vi "Init.vi"(8 "error in (no error)":errorcluster, 10 "Variant":variant, 11 "Avantes in":refnum<class "Avantes.lvclass">) -> (0 "error out":errorcluster, 3 "Avantes out":refnum<class "Avantes.lvclass">)   [LabVIEW 2020, in "Avantes.lvclass"]
uses:
  <instrlib>/Classes/CCD/Avantes/Avantes.lvclass
  <instrlib>/Classes/CCD/Avantes/Avantes.lvclass/Avantes.ctl
panel:
  out "Debug_Settings_Spectromter":string caption="Debug Spectromter"
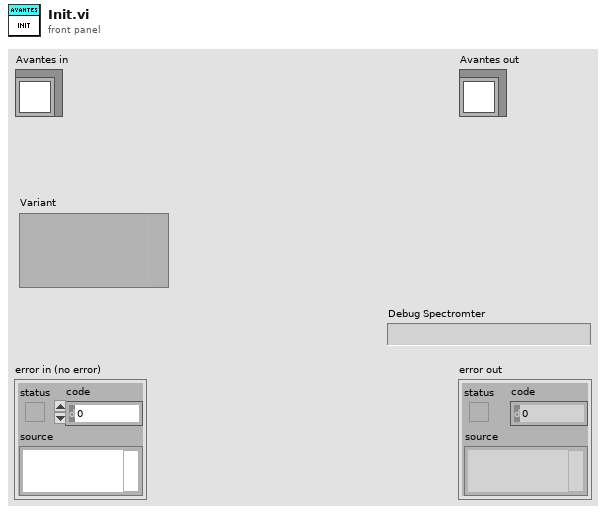
[diagram p1: front panel]
types:
  T1 = typedef "clusterdef.ctl" = cluster{"Len":u16, "ConfigVersion":u16, "UserFriendlyId":u8[], "DetectorType":cluster{"SensorType":u8, "NrPixels":u16, "Fit":sgl[], "NLEnable":u8, "NLCorrect":dbl[], "LowNLCounts":dbl, "HighNLCounts":dbl, "Gain":sgl[], "Reserved":sgl, "Offset":sgl[], "Extern Offset":sgl, "DefectivePixels":u16[]}, "IrradianceType":cluster{"SpectrumCalibrationType":cluster{"SmoothingType":cluster{"m_SmoothPix":u16, "SmoothModel":u8}, "CalInttime":sgl, "CalibConvers":sgl[]}, "CalibrationType":u8, "FiberDiameter":i32}, "SpectrumCalibrationType":cluster{"SmoothingType":cluster{"m_SmoothPix":u16, "SmoothModel":u8}, "CalInttime":sgl, "CalibConvers":sgl[]}, "SpectrumCorrectionType":sgl[], "StandAloneType":cluster{"StandAloneType":u8, "MeasConfigType":cluster{"StartPixel":u16, "StopPixel":u16, "IntegrationTime":sgl, "IntegrationDelay":u32, "NrAverages":u32, "DarkCorrectionType":cluster{"Enable CorDynDark":u8, "ForgetPercentage":u8}, "SmoothingType":cluster{"SmoothPix":u16, "SmoothModel":u8}, "SatDetection":u8, "TriggerType":cluster{"Trigger Mode":u8, "Trigger Source":u8, "Trigger SourceType":u8}, "ControlSettingsType":cluster{"StrobeControl":u16, "LaserDelay":u32, "LaserWidth":u32, "LaserWaveLength":sgl, "StoreToRam":u16}}, "Nmsr":i16}, "DynamicStorageType":cluster{"Nmsr":i32, "Reserved":u8[]}, "TempSensorType":sgl[], "TecControlType":cluster{"Enable":u8, "Setpoint":sgl, "Fit[NR_DAC_POL_COEF]":sgl[]}, "ProcessControlType":cluster{"AnalogLow":sgl[], "AnalogHigh":sgl[], "DigitalLow":sgl[], "DigitalHigh":sgl[]}, "EthernetSettingsType":cluster{"IpAddr":u32, "NetMask":u32, "Gateway":u32, "DhcpEnabled":u8, "TcpPort":u16, "LinkStatus":u8}, "Reserved":u8[], "OemData":u8[]}
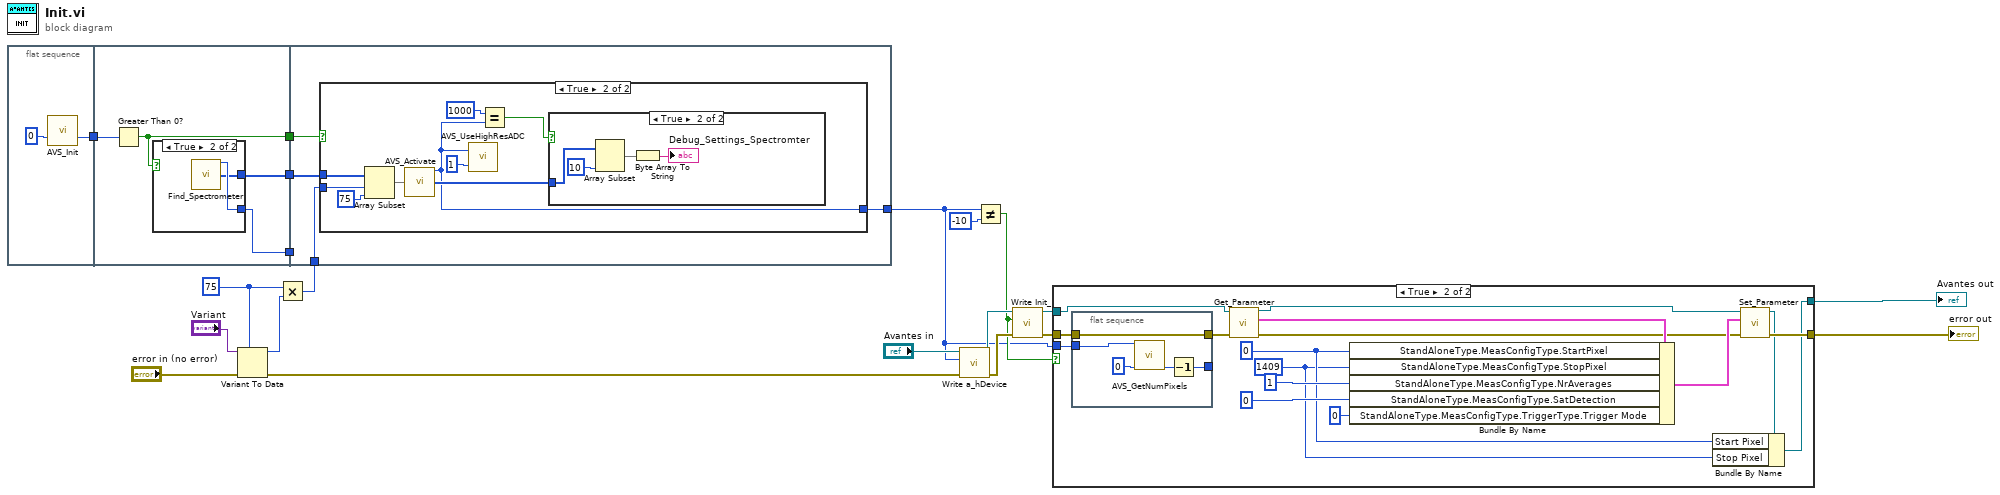
[diagram p0: block diagram]
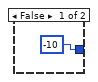
[diagram p4: hidden frame]
diagram:
  w11 = 75 ("length")
  n1 = flat-sequence {
    tunnel: [w21] -> w20
    tunnel: w20 -> [w26]
    tunnel: [w25] -> w19
    tunnel: [w24] -> w18
    tunnel: [w23] -> w17
    tunnel: w19 -> [_]
    tunnel: w18 -> [w32]
    tunnel: [w31] -> w1
    tunnel: w17 -> [w30]
    tunnel: w10 -> [w29]
    frame #0 {
      n2 = call <instrlib>:"AVS_Init.vi"("a_Port"=0) -> ("Output Value"=w21:i32)  [unwired: 14 in]
    }
    frame #1 {
      n3 = Greater Than 0?(x=w26) -> (x > 0?=w23:bool)
      n4 = case shown="True" w23 {
        tunnel: [_ w28] -> w25
        tunnel: [_ w27] -> w24
        frame False {
        }
        frame True {
          n5 = call <instrlib>:"Find_Spectrometer.vi"() -> ("NrOfDevices"=w28:i32, "AviableSpec"=w27:u8[])  [unwired: 14 in]
        }
      }
    }
    frame #2 {
      n6 = case shown="True" w30 {
        tunnel: w32 -> [_ w42]
        tunnel: [-10 ("Output Value") w35] -> w31
        tunnel: w29 -> [_ w36]
        frame False {
        }
        frame True {
          n7 = Array Subset(array=w42, index=w36, length=75) -> (w40:u8[])
          n8 = call <instrlib>:"AVS_Activate.vi"("a_pDeviceId"=w40) -> ("Output Value"=w35:i32, "a_pDeviceId"=w37:u8[])  [unwired: 13 in]
          n9 = call <instrlib>:"AVS_UseHighResADC.vi"("a_Enable"=u8 1, "a_hDevice"=w35) -> ()  [unwired: 1 out]
          n10 = Equal?(x=1000, y=w35) -> (x = y?=w38:bool)
          n11 = case shown="True" w38 {
            tunnel: w37 -> [_ w46]
            frame False {
            }
            frame True {
              n12 = Array Subset(array=w46, length=10) -> (w44:u8[])  [unwired: 1 in]
              n13 = Byte Array To String(unsigned byte array=w44) -> (string=→"Debug_Settings_Spectromter":string)
            }
          }
        }
      }
    }
  }
  n14 = Variant To Data(error in="error in (no error)", type=w11, Variant="Variant") -> (data=w12:i32, error out=w13:errorcluster)
  n15 = Multiply(x=w11, y=w12) -> (x*y=w10:i32)
  n16 = call-dynamic "Write a_hDevice.vi"("error in (no error)"=w13, "a_hDevice"=w1, "Avantes in"="Avantes in") -> ("error out"=w7:errorcluster, "Avantes out"=w8:refnum<class "Avantes.lvclass">)  [unwired: 7 in]
  n17 = Not Equal?(x=w1, y=-10) -> (x != y?=w4:bool)
  n18 = call-dynamic "Write Init_.vi"("error in (no error)"=w7, "Init?"=w4, "Avantes in"=w8) -> ("error out"=w6:errorcluster, "Avantes out"=w5:refnum<class "Avantes.lvclass">)  [unwired: 7 in]
  n19 = case shown="True" w4 {
    tunnel: w6 -> [w47 w60]
    tunnel: w5 -> [w48 w64]
    tunnel: [w47 w58] -> w3
    tunnel: [w48 w50] -> w2
    tunnel: w1 -> [_ w61]
    frame False {
    }
    frame True {
      w51 = u16 1409 ("StopPixel")
      w52 = u16 0 ("StartPixel")
      n20 = flat-sequence {
        tunnel: w61 -> [w68]
        tunnel: w60 -> [w67]
        tunnel: [w67] -> w59
        tunnel: [w65] -> _
        frame #0 {
          n21 = call <instrlib>:"AVS_GetNumPixels.vi"("a_hDevice"=w68, "a_pNumPixels"=u16 0) -> ("a_pNumPixels"=w66:u16)  [unwired: 12 in, 1 out]
          n22 = Decrement(x=w66) -> (x-1=w65:u16)
        }
      }
      n23 = call-dynamic "Get_Parameter.vi"("error in (no error)"=w59, "Avantes in"=w64) -> ("error out"=w54:errorcluster, "DeviceConfig"=w56:T1, "Avantes out"=w57:refnum<class "Avantes.lvclass">)  [unwired: 7 in]
      n24 = Bundle By Name(cluster=w56, "StandAloneType.MeasConfigType.StartPixel"=w52, "StandAloneType.MeasConfigType.StopPixel"=w51, "StandAloneType.MeasConfigType.NrAverages"=u32 1 ("NrAverages"), "StandAloneType.MeasConfigType.SatDetection"=u8 0 ("SatDetection"), "StandAloneType.MeasConfigType.TriggerType.Trigger Mode"=u8 0) -> (w55:T1)
      n25 = call-dynamic "Set_Parameter.vi"("error in (no error)"=w54, "DeviceConfig"=w55, "Avantes in"=w57) -> ("error out"=w58:errorcluster, "Avantes out"=w53:refnum<class "Avantes.lvclass">)  [unwired: 7 in]
      n26 = Bundle By Name(cluster=w53, "Start Pixel"=w52, "Stop Pixel"=w51) -> (w50:refnum<class "Avantes.lvclass">)
    }
  }
  "error out" <- w3
  "Avantes out" <- w2
